vi "ConfigInputMix.vi"(1 "MulticolumnListbox in":refnum<vi>, 3 "ItemNames in":string[][](array[string])) -> (0 "ItemNames out":string[][](array[string]))   [LabVIEW 2018, in "Config.lvlib"]
uses:
  Config.lvlib
panel:
  in  "Replace":bool
  in  "Insert":bool
  in  "Append":bool
  in  "Mixing Cycles":dbl=4.0 min=4.0 step=1.0
  in  "Mixing Time":dbl=1.0 min=1.0 step=1.0 format="%<%H:%M:%S>t"
  # "Mixing Step"
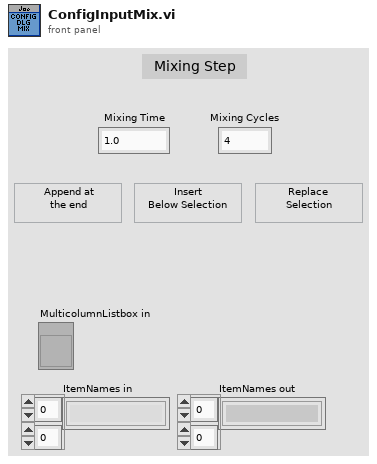
[diagram p1: front panel]
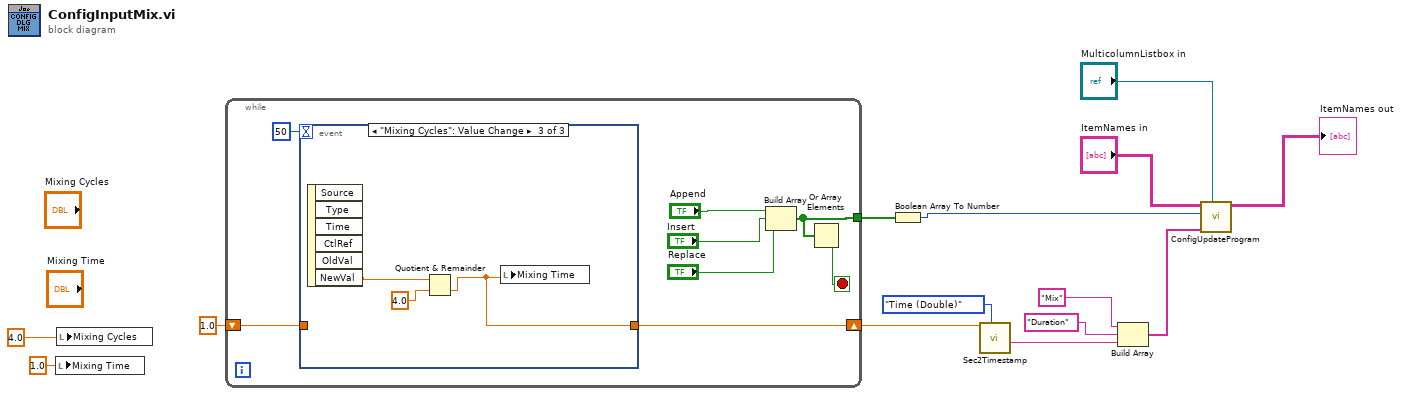
[diagram p0: block diagram]
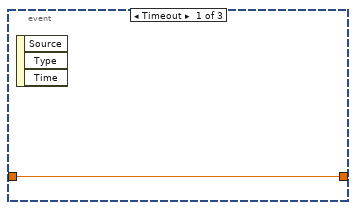
[diagram p2: hidden frame]
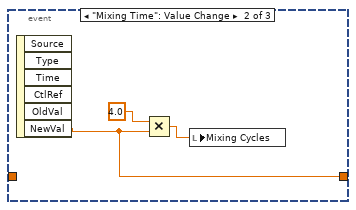
[diagram p3: hidden frame]
diagram:
  n1 = local write "Mixing Time"(1.0 ("Mixing Time")) -> ()
  n2 = local write "Mixing Cycles"(4.0 ("Mixing Cycles")) -> ()
  n3 = while {
    tunnel: [w17] -> w13
    shift-right: [w16] -> w7
    shift-left: 1.0 ("NewVal") -> [w15]
    stop <- w18 stop-if-true
    n4 = event shown="[2] \"Mixing Cycles\": Value Change" {
      selector: _ -> [_ _ _]
      dyn-events: _ -> [_ _ _]
      timeout: 50 -> [_ _ _]
      tunnel: [w23 w24 w27] -> w16
      tunnel: w15 -> [w23 _ _]
      event Timeout {
        n5 = event-data() -> ()  [unwired: 1 in, 3 out]
      }
      event "Mixing Time": Value Change {
        n6 = event-data() -> ("NewVal"=w24:dbl)  [unwired: 1 in, 5 out]
        n7 = Multiply(x=4.0, y=w24) -> (x*y=w25:dbl)
        n8 = local write "Mixing Cycles"(w25) -> ()
      }
      event "Mixing Cycles": Value Change {
        n9 = event-data() -> ("NewVal"=w28:dbl)  [unwired: 1 in, 5 out]
        n10 = Quotient & Remainder(x=w28, y=4.0) -> (floor(x/y)=w27:dbl)  [unwired: 1 out]
        n11 = local write "Mixing Time"(w27) -> ()
      }
    }
    n12 = Build Array("Append", "Insert", "Replace") -> (w17:bool[])
    n13 = Or Array Elements(Boolean array=w17) -> (logical OR=w18:bool)
  }
  n14 = Boolean Array To Number(Boolean array=w13) -> (number=w5:u32)
  n15 = call "Sec2Timestamp.vi"("Input Selection"=enum32{"Time (Double)", "Time (Time Stamp)"}."Time (Double)", "Input Time (Double)"=w7) -> ("date/time string"=w10:string)  [unwired: 7 in, 2 out]
  n16 = Build Array("Mix", "Duration", w10) -> (w6:string[])
  n17 = call "ConfigUpdateProgram.vi"("MulticolumnListbox in"="MulticolumnListbox in", "New Element"=w6, "Operation"=w5, "ItemNames in"="ItemNames in") -> ("ItemNames out"=→"ItemNames out":string[][])  [unwired: 7 in]
